vi "ExecuteTask.vi"(8 "error in (no error)":errorcluster caption="错误输入（无错误）", 11 "Task":enum16{"Task A", "Task B", "Task C"}(ring)) -> (0 "error out":errorcluster caption="错误输出")   [LabVIEW 2013]
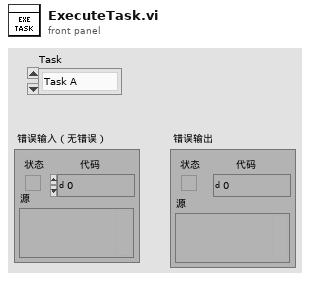
[diagram p1: front panel]
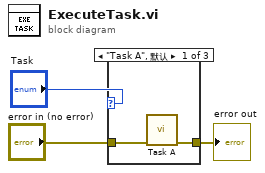
[diagram p0: block diagram]
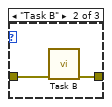
[diagram p2: hidden frame]
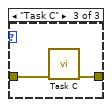
[diagram p3: hidden frame]
diagram:
  n1 = case shown="\"Task A\", 默认" "Task" {
    tunnel: "error in (no error)" -> [w5 w7 w9]
    tunnel: [w4 w6 w8] -> w1
    frame "Task A", Default {
      n2 = call "Task A.vi"("error in (no error)"=w5) -> ("error out"=w4:errorcluster)  [unwired: 10 in]
    }
    frame "Task B" {
      n3 = call "Task B.vi"("error in (no error)"=w7) -> ("error out"=w6:errorcluster)  [unwired: 10 in]
    }
    frame "Task C" {
      n4 = call "Task C.vi"("error in (no error)"=w9) -> ("error out"=w8:errorcluster)  [unwired: 10 in]
    }
  }
  "error out" <- w1
